vi "Random String.vi"() -> (3 "string":string)   [LabVIEW 2017, in "Unit Tests.lvlib"]
uses:
  Unit Tests.lvlib
  <vilib>/Analysis/NI_AALBase.lvlib
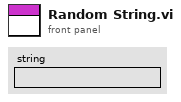
[diagram p1: front panel]
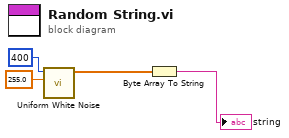
[diagram p0: block diagram]
diagram:
  n1 = call <vilib>:"Uniform White Noise.vi"("amplitude"=255.0, "samples"=400) -> ("uniform white noise"=w3:dbl[])  [unwired: 8 in, 1 out]
  n2 = Byte Array To String(unsigned byte array=w3) -> (string=→"string":string)
